vi "IT6522D_Measure.vi"(8 "error in":errorcluster caption="错误输入（无错误）", 9 "等待时间(毫秒)":u32=100, 10 "Measure":enum16{"MEASure:CURRent?", "MEASure:VOLTage?"}(ring), 11 "MyIndex":u8) -> (0 "error out":errorcluster, 3 "数值":dbl)   [LabVIEW 2015, in "IT6522D.lvlib"]
uses:
  IT6522D.lvlib
  <vilib>/Instr/_visa.llb/VISA Configure Serial Port (Instr).vi
panel:
  out "VISA":refnum<visa-resource-name>
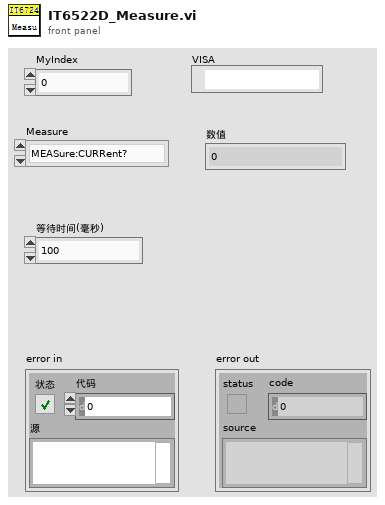
[diagram p1: front panel]
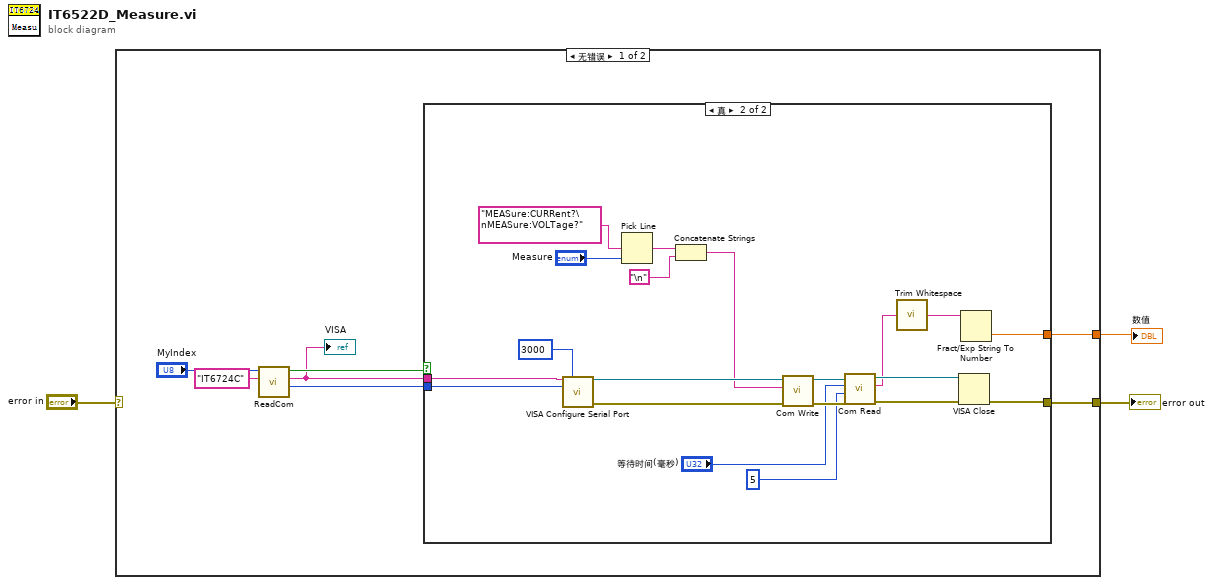
[diagram p0: block diagram]
diagram:
  n1 = case shown="无错误" "error in" {
    selector: "error in" -> [_ w31]
    tunnel: [w10 w31] -> w3
    tunnel: [w4 _] -> w1
    frame No Error {
      n2 = call "ReadCom.vi"("仪器名称"="IT6724C", "MyIndex"="MyIndex") -> ("Baudrate"=w5:i32, "COM"=w6:string, "OK?"=w7:bool)  [unwired: 7 in]
      "VISA" <- w6
      n3 = case shown="真" w7 {
        tunnel: [_ w30] -> w10
        tunnel: w6 -> [_ w29]
        tunnel: w5 -> [_ w28]
        tunnel: [_ w11] -> w4
        frame False {
        }
        frame True {
          n4 = call-poly "VISA Configure Serial Port"("VISA resource name"=w29, "timeout (10sec)"=u32 3000, "baud rate (9600)"=w28) -> ("VISA resource name out"=w26:refnum<visa-resource-name>, "error out"=w25:errorcluster)  [unwired: 11 in]
          n5 = Pick Line(multi-line string="MEASure:CURRent?\nMEASure:VOLTage?", line index="Measure") -> (output string=w18:string)  [unwired: 1 in]
          n6 = Concatenate Strings(w18, "\n") -> (w14:string)
          n7 = call "Com Write.vi"("错误输入（无错误）"=w25, "Wbuff"=w14, "VISA In"=w26) -> ("错误输出"=w23:errorcluster, "VISA Out"=w24:refnum<visa-resource-name>)  [unwired: 7 in]
          n8 = call "Com Read.vi"("错误输入（无错误）"=w23, "num"=u32 5, "超时"="等待时间(毫秒)", "VISA In"=w24) -> ("错误输出"=w22:errorcluster, "buff"=w13:string, "VISA Out"=w21:refnum<visa-resource-name>)  [unwired: 5 in]
          n9 = call <vilib>:"Trim Whitespace.vi"("string"=w13) -> ("trimmed string"=w12:string)  [unwired: 1 in]
          n10 = VISA Close(VISA resource name=w21, error in (no error)=w22) -> (error out=w30:errorcluster)
          n11 = Fract/Exp String To Number(string=w12) -> (number=w11:dbl)  [unwired: 3 in, 1 out]
        }
      }
    }
    frame Error {
    }
  }
  "数值" <- w1
  "error out" <- w3
